vi "setReg.vi"(7 "I2C Channel":u8, 8 "error in":errorcluster, 9 "Data":u8[](array[numeric]), 10 "I2C Slave Address":u8 format="%.0x", 11 "LINX Resource in":T1) -> (0 "error out":errorcluster, 3 "LINX Resource":T1)   [LabVIEW 2014]
uses:
  <vilib>/MakerHub/LINX/Private/Type Defs/LINX Ref.ctl
  <vilib>/MakerHub/LINX/Private/Type Defs/Platform.ctl
  <vilib>/MakerHub/LINX/Private/Type Defs/Interface.ctl
  <vilib>/MakerHub/LINX/Private/Device/Type Defs/LINX Device Config.ctl
  <vilib>/MakerHub/LINX/Private/Device/Type Defs/TCP Config.ctl
  <vilib>/MakerHub/LINX/Private/Device/Type Defs/Channels.ctl
  <vilib>/myRIO/Instrument Drivers/Onboard IO/I2C/typedefs/I2C User Configuration.ctl
  <vilib>/myRIO/Instrument Drivers/Onboard IO/I2C/typedefs/I2C Transfer Rate.ctl
  <vilib>/Utility/error.llb/Error Cluster From Error Code.vi
  <vilib>/myRIO/Common/Instrument Driver Framework/myRIO v1.0/I2C/vis/myRIO v1.0 Configure I2C.vi
  <vilib>/myRIO/Common/Instrument Driver Framework/myRIO v1.0/I2C/vis/myRIO v1.0 Write I2C.vi
  <vilib>/myRIO/Instrument Drivers/Onboard IO/I2C/I2C.lvlib
  <vilib>/MakerHub/LINX/LMH-LINX.lvlib
  <vilib>/MakerHub/LINX/Private/Device/Device.lvlib
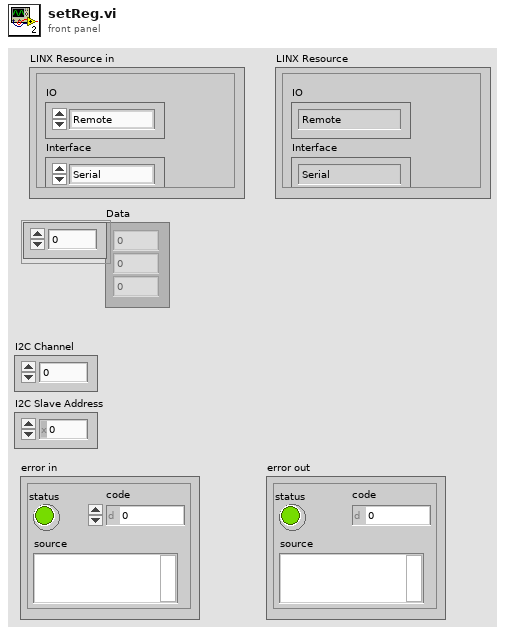
[diagram p1: front panel]
types:
  T1 = typedef "LMH-LINX.lvlib/LINX Ref.ctl" = cluster{"IO":T2, "Interface":T3, "LINX Device Config":T4}
  T2 = typedef "LMH-LINX.lvlib/Platform.ctl" = enum16{"Remote", "Local"}
  T3 = typedef "LMH-LINX.lvlib/Interface.ctl" = enum16{"Serial", "TCP"}
  T4 = typedef "LMH-LINX.lvlib/Device.lvlib/LINX Device Config.ctl" = cluster{"Interface":T3, "COM Port":refnum<visa-resource-name>, "TCP Configuration":T5, "Device Family":u8, "Device ID":u8, "Device Name":string, "TCP Ref":refnum<k5>, "Channels":T6}
  T5 = typedef "LMH-LINX.lvlib/Device.lvlib/TCP Config.ctl" = cluster{"IP Address":string, "Port":u16}
  T6 = typedef "LMH-LINX.lvlib/Channels.ctl" = cluster{"DI":u8[], "DO":u8[], "AI":u8[], "AO":u8[], "PWM":u8[], "QE":u8[], "UART":u8[], "I2C 2":u8[], "SPI":u8[], "CAN":u8[], "Servo":u8[], "AI Ref (V)":dbl, "AI Resolution (Bits)":u8, "AO Ref (V)":dbl, "AO Resolution (Bits)":u8}
  T7 = typedef "I2C.lvlib/I2C User Configuration.ctl" = cluster{"I2C Transfer Rate":T8}
  T8 = typedef "I2C.lvlib/I2C Transfer Rate.ctl" = enum16{"Standard mode (100 kbps)", "Fast mode (400 kbps)"}
  T9 = typedef "I2C.lvlib/I2C Reference.ctl" = cluster{"myRIO Reference":T10, "I2C Channels Enum":T14, "I2C Configuration":T15}
  T10 = typedef "myRIO Generic Hardware Reference.ctl" = cluster{"myRIO Model":T11, "myRIO Hardware Reference":T12}
  T11 = typedef "Hardware Version Enum.ctl" = enum16{"Unknown", "myRIO-1900", "myRIO-1950"}
  T12 = typedef "myRIO v1.0 Reference.ctl" = cluster{"Generic FPGA Reference":T13, "Allow multiple opens":bool}
  T13 = typedef "Generic FPGA Reference.ctl" = refnum<k20>
  T14 = typedef "I2C Channels Enum.ctl" = enum16{"Not Connected", "A/I2C", "B/I2C"}
  T15 = typedef "I2C.lvlib/I2C Configuration.ctl" = cluster{"I2C Transfer Rate":T8}
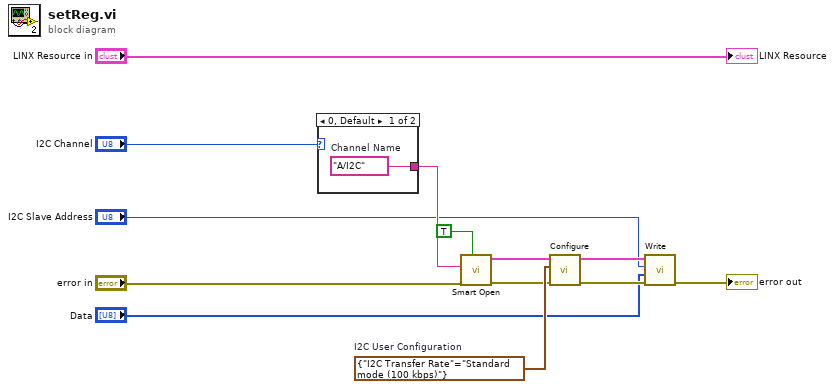
[diagram p0: block diagram]
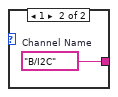
[diagram p2: hidden frame]
diagram:
  w13 = T7 {"I2C Transfer Rate"=enum."Standard mode (100 kbps)"}  # I2C User Configuration
  n1 = case shown="0, Default" "I2C Channel" {
    tunnel: [w14 w15] -> w8
    frame 0, Default {
      w14 = tag "A/I2C"  # Channel Name
    }
    frame 1 {
      w15 = tag "B/I2C"  # Channel Name
    }
  }
  n2 = call <vilib>:"Smart Open.vi"("Allow multiple opens?"=TRUE, "error in (no error)"="error in", "Channel Name"=w8) -> ("error out"=w11:errorcluster, "I2C Ref Out"=w12:T9)  [unwired: 7 in]
  n3 = call <vilib>:"Configure.vi"("error in (no error)"=w11, "I2C User Configuration"=w13, "I2C Ref In"=w12) -> ("error out"=w9:errorcluster, "I2C Ref Out"=w10:T9)  [unwired: 7 in]
  n4 = call <vilib>:"Write.vi"("error in (no error)"=w9, "Bytes to Write"="Data", "Slave Address (7-bit)"="I2C Slave Address", "I2C Ref In"=w10) -> ("error out"=→"error out":errorcluster)  [unwired: 6 in, 1 out]
  "LINX Resource" <- "LINX Resource in"
